vi "Run FPGATarget2.vi"(6 "clone#":i32, 11 "session":u32) -> ()   [LabVIEW 2020, in "NI_TargetHelper.lvlib"]
uses:
  <vilib>/TargetSupport/NI_TargetHelper/NI_TargetHelper.lvlib
  NiFpgaLv.dll
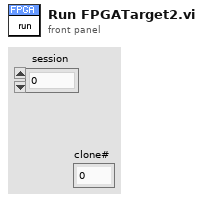
[diagram p1: front panel]
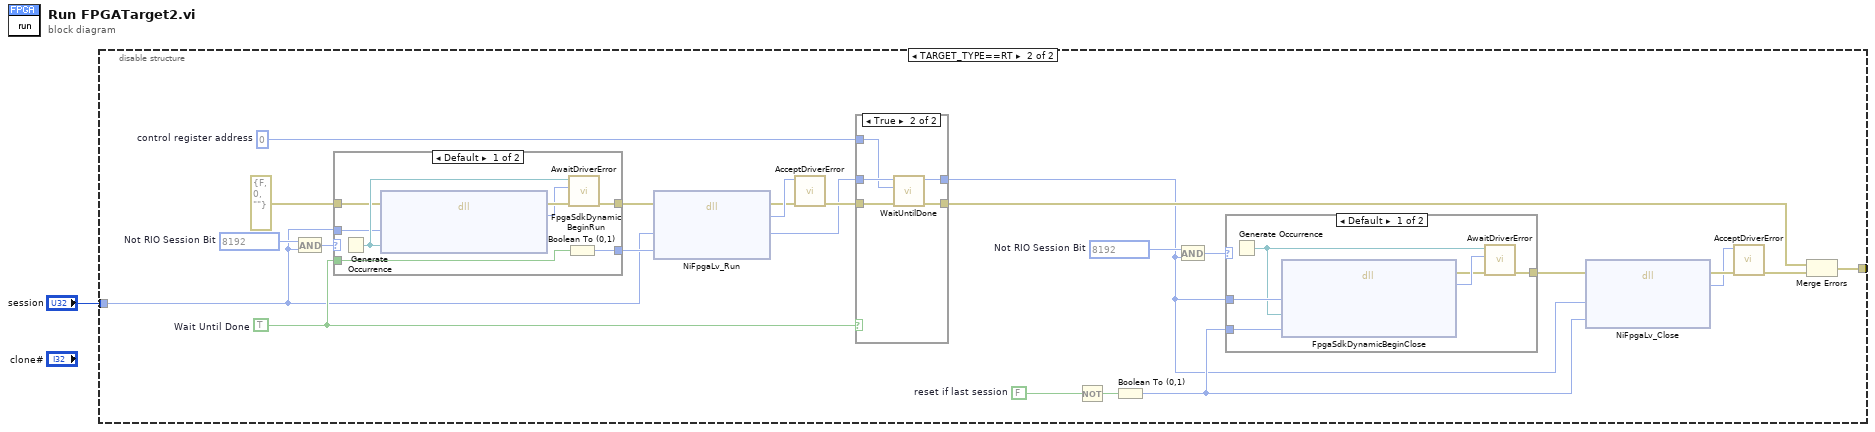
[diagram p0: block diagram]
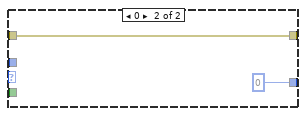
[diagram p3: hidden frame]
diagram:
  n1 = disable-structure shown="TARGET_TYPE==RT" {
    disable-tunnel: "session" -> [_ w14]
    disable-tunnel: [_ w2] -> _
    frame condition #0 (active) {
    }
    frame condition #1 {
      w6 = FALSE  # reset if last session
      w5 = u32 8192  # Not RIO Session Bit
      w15 = u32 0  # control register address
      w16 = u32 8192  # Not RIO Session Bit
      w17 = TRUE  # Wait Until Done
      n2 = And(x=w16, y=w14) -> (x .and. y?=w24:u32)
      n3 = case shown="Default" w24 {
        tunnel: errorcluster {"status"=FALSE, "code"=0, "source"=""} ("error in") -> [w30 w35]
        tunnel: [w29 w35] -> w23
        tunnel: w14 -> [w28 _]
        tunnel: w17 -> [w27 _]
        tunnel: [w26 u32 0 ("attribute")] -> w25
        frame Default {
          n4 = Generate Occurrence() -> (w33:refnum<k4>)
          n5 = dll-call lib="LabVIEW" fn="FpgaSdkDynamicBeginRun"(error in=w30, "session"=w28, "occurrence"=w33) -> (error out=w32:errorcluster, "status"=w31:i32)  [unwired: 4 in, 1 out]
          n6 = Boolean To (0,1)(Boolean=w27) -> (0, 1=w26:i16)
          n7 = call <vilib>:"AwaitDriverError.vi"("error in (no error)"=w32, "status"=w31, "Occurrence in"=w33) -> ("error out"=w29:errorcluster)  [unwired: 8 in]
        }
        frame 0 {
        }
      }
      n8 = dll-call lib="NiFpgaLv.*" fn="NiFpgaLv_Run" label="niLvFpgaRun"(error in=w23, "sessionID"=w14, "attribute"=w25) -> (error out=w19:errorcluster, "status"=w20:i32, "sessionID"=w18:u32)  [unwired: 3 in, 1 out]
      n9 = call <vilib>:"AcceptDriverError.vi"("error in (no error)"=w19, "status"=w20) -> ("error out"=w21:errorcluster)  [unwired: 9 in]
      n10 = case shown="True" w17 {
        tunnel: w18 -> [w37 w39]
        tunnel: [w36 w42] -> w4
        tunnel: w15 -> [_ w38]
        tunnel: w21 -> [w36 w41]
        tunnel: [w37 w40] -> w3
        frame False {
        }
        frame True {
          n11 = call <vilib>:"WaitUntilDone.vi"("error in (no error)"=w41, "control register address"=w38, "sessionID in"=w39) -> ("error out"=w42:errorcluster, "sessionID out"=w40:u32)  [unwired: 7 in]
        }
      }
      n12 = Not(x=w6) -> (.not. x?=w7:bool)
      n13 = Boolean To (0,1)(Boolean=w7) -> (0, 1=w13:i16)
      n14 = And(x=w5, y=w3) -> (x .and. y?=w8:u32)
      n15 = case shown="Default" w8 {
        tunnel: [w44 _] -> w9
        tunnel: w3 -> [w48 _]
        tunnel: w13 -> [w47 _]
        frame Default {
          n16 = Generate Occurrence() -> (w43:refnum<k4>)
          n17 = dll-call lib="LabVIEW" fn="FpgaSdkDynamicBeginClose"("session"=w48, "occurrence"=w43, "noResetIfLastSession"=w47) -> (error out=w45:errorcluster, "status"=w46:i32)  [unwired: 6 in, 1 out]
          n18 = call <vilib>:"AwaitDriverError.vi"("error in (no error)"=w45, "status"=w46, "Occurrence in"=w43) -> ("error out"=w44:errorcluster)  [unwired: 8 in]
        }
        frame 0 {
        }
      }
      n19 = dll-call lib="NiFpgaLv.*" fn="NiFpgaLv_Close" label="niLvFpgaClose"(error in=w9, "sessionID"=w3, "noResetIfLastSession"=w13) -> (error out=w11:errorcluster, "status"=w10:i32)  [unwired: 3 in, 2 out]
      n20 = call <vilib>:"AcceptDriverError.vi"("error in (no error)"=w11, "status"=w10) -> ("error out"=w12:errorcluster)  [unwired: 9 in]
      n21 = Merge Errors(w4, w12) -> (w2:errorcluster)
    }
  }
